vi "DésV2.vi"() -> ()   [LabVIEW 2018]
panel:
  in  "Numeric":u32=1 min=1 max=7
  out "led 1":bool
  out "led 3":bool
  out "led 2":bool
  out "led 6":bool
  out "led 4":bool
  out "led 5":bool
  out "led7":bool
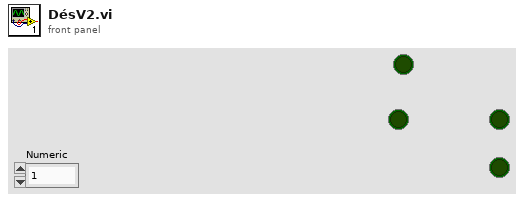
[diagram p1: front panel]
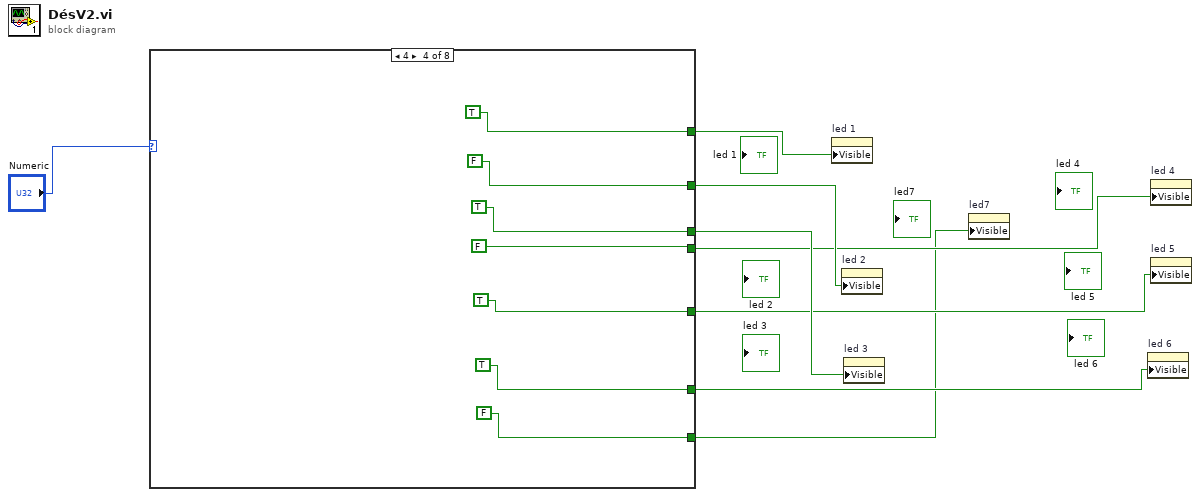
[diagram p0: block diagram]
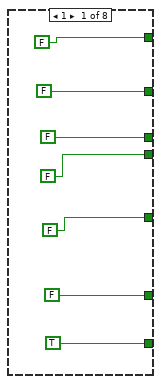
[diagram p2: hidden frame]
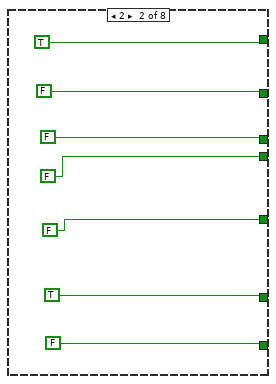
[diagram p3: hidden frame]
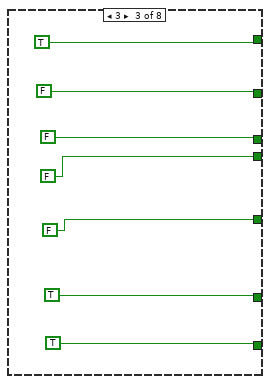
[diagram p4: hidden frame]
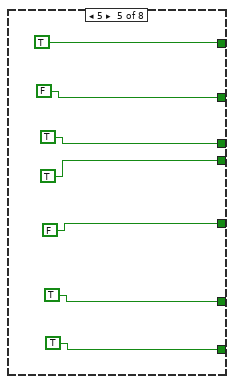
[diagram p5: hidden frame]
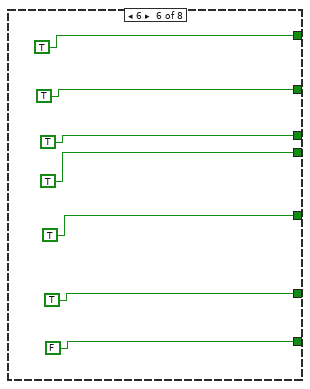
[diagram p6: hidden frame]
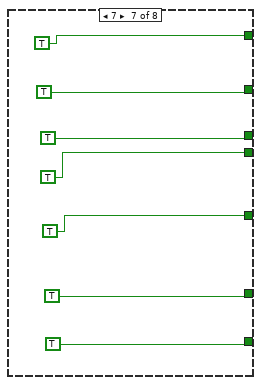
[diagram p7: hidden frame]
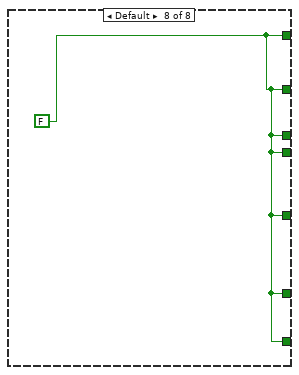
[diagram p8: hidden frame]
diagram:
  n1 = case shown="4" "Numeric" {
    tunnel: [FALSE TRUE TRUE TRUE TRUE TRUE TRUE w58] -> w8
    tunnel: [FALSE FALSE FALSE FALSE FALSE TRUE TRUE w58] -> w7
    tunnel: [FALSE FALSE FALSE TRUE TRUE TRUE TRUE w58] -> w6
    tunnel: [FALSE FALSE FALSE FALSE TRUE TRUE TRUE w58] -> w5
    tunnel: [FALSE FALSE FALSE TRUE FALSE TRUE TRUE w58] -> w4
    tunnel: [FALSE TRUE TRUE TRUE TRUE TRUE TRUE w58] -> w3
    tunnel: [TRUE FALSE TRUE FALSE TRUE FALSE TRUE w58] -> w2
    frame 1 {
    }
    frame 2 {
    }
    frame 3 {
    }
    frame 4 {
    }
    frame 5 {
    }
    frame 6 {
    }
    frame 7 {
    }
    frame Default {
      w58 = FALSE
    }
  }
  n2 = property on="led 1" class="Bool (strict)"("Visible"=w8) -> ()  [unwired: 2 in, 2 out]
  n3 = property on="led 2" class="Bool (strict)"("Visible"=w7) -> ()  [unwired: 2 in, 2 out]
  n4 = property on="led 3" class="Bool (strict)"("Visible"=w6) -> ()  [unwired: 2 in, 2 out]
  n5 = property on="led7" class="Bool (strict)"("Visible"=w2) -> ()  [unwired: 2 in, 2 out]
  n6 = property on="led 6" class="Bool (strict)"("Visible"=w3) -> ()  [unwired: 2 in, 2 out]
  n7 = property on="led 4" class="Bool (strict)"("Visible"=w5) -> ()  [unwired: 2 in, 2 out]
  n8 = property on="led 5" class="Bool (strict)"("Visible"=w4) -> ()  [unwired: 2 in, 2 out]
